vi "Example IRQ 1.vi"(8 "Error In":errorcluster) -> (0 "Error Out":errorcluster)   [LabVIEW 2014]
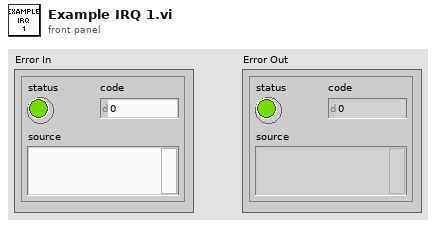
[diagram p1: front panel]
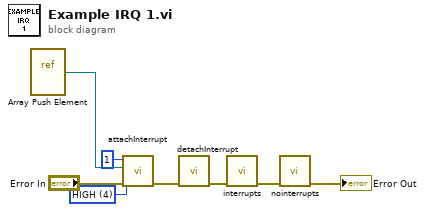
[diagram p0: block diagram]
diagram:
  w1 = u16 4 items=["LOW", "CHANGE", "RISING", "FALLING", "HIGH"] ("mode")
  n1 = vi-ref "Array Push Element.vi"() -> (w3:refnum<vi>)
  n2 = call "attachInterrupt.vi"("Error In"="Error In", "mode"=w1, "VI Refnum"=w3, "pin number"=1) -> ("Error Out"=w7:errorcluster)  [unwired: 7 in]
  n3 = call "detachInterrupt.vi"("Error In"=w7) -> ("Error Out"=w6:errorcluster)  [unwired: 10 in]
  n4 = call "interrupts.vi"("Error In"=w6) -> ("Error Out"=w5:errorcluster)  [unwired: 10 in]
  n5 = call "nointerrupts.vi"("Error In"=w5) -> ("Error Out"=→"Error Out":errorcluster)  [unwired: 10 in]
